vi "Exercise introduction.vi"(5 "Exercise Execution Mode":T2, 6 "Numero USP":dbl format="%#.13f", 7 "Exercise Number":T1, 8 "Error In":errorcluster, 9 "Waveform In":waveform(dbl), 10 "Array":bool[](array[boolean]), 11 "Exercise Folder Path":path) -> (0 "Error Out":errorcluster, 1 "Waveform Out":waveform(dbl), 2 "Done":dbl)   [LabVIEW 2014]
uses:
  Ctls/teval.ctl
  Ctls/t1q1.ctl
  Ctls/t1q2.ctl
  Ctls/ExerciseState.ctl
  Ctls/ExerciseNumeration.ctl
  <vilib>/Utility/miscctls.llb/LVPointTypeDef.ctl
  Ctls/radiobutton010.ctl
panel:
  out "Exercise Tab":T3(tab)
  in  "Close 3":bool
  in  "TEVAL":T4 caption="Perguntas"
  in  "Close":bool
  in  "T1E1":T5 {"C (F)" format="%#_9f"}
  in  "Close 2":bool
  in  "T1E2":T6 caption="Dado o sinal ao lado (presente no painel principal do exercício), faça uso das ferramentas até agora fornecidas para indicar:" {"C (F)" format="%#_9f"}
  # "PSI3214\nLaboratório de Instrumentação Elétrica"
  # "Avaliação do Tutorial"
  # "Ao longo do tutorial foram utilizados materiais em PDF para referência do aluno, materiais em vídeo para acompanhamento mais dinâmico. Neste questionário serão avaliados alguns parâmetros quantitativos a fim de se melhorar a qualidade dos tutoriais fornecidos ao longo dos anos. É importante deixar claro que não será pedida nenhuma informação que possa identificar o aluno, de modo a preservar a privacidade de cada um."
  # "AA.1) Em relação ao Material Escrito disponibilizado em PDF, avalie:"
  # "Muito Pequeno"
  # "Muito Grande"
  # "Pouco Tempo"
  # "Muito Tempo"
  # "Conteúdo do tutorial\npouco adequado às aulas"
  # "Conteúdo do tutorial\nbem adequado às aulas"
  # "Conteúdo do tutorial\nfoi pouco claro/coeso"
  # "Conteúdo do tutorial\nfoi bem claro/coeso"
  # "Tutorial atuou muito mal\ncomo reforço das aulas"
  # "Tutorial atuou muito bem \ncomo reforço das aulas"
  # "Problemas pouco\ncontextualizados"
  # "Problemas muito bem\ncontextualizados"
  # "Ferramentas pouco\ncontextualizadas"
  # "Ferramentas muito bem\ncontextualizadas"
  # "Foi de pouca ajuda na compreensão\nde outras materias"
  # "Foi de grande ajuda na compreensão\nde outras materias"
  # "AA.2) Em relação ao sua compreensão do tutorial, realize uma auto-avaliação sobre sua:"
  # "não compreendi nenhum tópico\nde programação apresentada"
  # "compreendi completamente\ntoda programação apresentada"
  # "não compreendi nenhum tópico\nde teoria apresentada"
  # "compreendi completamente\ntoda teoria apresentada"
  # "não compreendi nenhuma das\nproblemáticas apresentadas"
  # "compreendi completamente\ntodas as problemáticas apresentadas"
  # "PSI3214\nLaboratório de Instrumentação Elétrica"
  # "Exercício 1.1\nCircuito RC/RL"
  # "Como primeiro exercício, vamos rever como calcular parâmetros essênciais em circuitos RL/RC. Neste exercício será apresentado um circuito RL ou RC, cabe ao aluno a identificação de qual circuito se trata e como realizar os calculos dos parâmetros pedidos."
  # "Fig. 1.1 - Circuito RC"
  # "Fig. 1.2 - Circuito RL"
  # "Utilize o sinal gerado no VI [Exercicio 1.vi] para responder as perguntas abaixo:"
  # "Para fechar a tela do enunciado, pressione o botão \"Close Form\""
  # "A) Analise o sinal dado e indique:"
  # "B) Considerando as equações utilizadas para simulação de circuitos RC ou RL, dê os valores de:"
  # "PSI3214\nLaboratório de Instrumentação Elétrica"
  # "Exercício 1.2\nAcelerômetro MEMS"
  # "Até o presente momento foi realizada uma apresentação de programação em LabVIEW em vias de simular um circuito RC/RL. Na prática tal tarefa não seria de muito interesse para uma empresa. Vamos agora utilizar o ambiente LabVIEW para contextualizar a utilização de Circuitos RC/RL na industria:"
  # "Para fechar a tela do enunciado, pressione o botão \"Close Form\""
  # "Um dos grandes avanços na área de engenharia Mecânica e Elétrica das ultimas décadas é o advento das tecnologias MEMS (Sistemas Microeletromecânicos), que nos permitiu a construção de polias, engrenagens e motores em escala microscópica. Dentre algumas das microestruturas construídas podemos destacar os Acelerômetros MEMS, os quais permitiram a construção de celulares com capacidade de localização 3D, até sistemas de misseis teleguiados.\n    Vamos focar neste exercício no princípio fundamental que permite o funcionamento de um Acelerômetro MEMS. A estrutura é composta, basicamente, de um capacitor variavel. Conforme uma força é aplicada ao sensor, o eletrodo móvel se aproxima ou afasta do eletrodo fixo. Deste modo, ao medirmos a capacitância do dispositivo, mediremos indiretamente a força a ele aplicada.\n    Dentre os inúmeros modos que podemos identificar a capacitância de um circuito RC, iremos fazer uso aquele que foi utilizado ao longo do tutorial."
  # "A) Descreva o sinal de controle utilizado no sistema:"
  # "B) Com base no gráfico de corrente, indique qual a Resistência do dispositivo MEMS:"
  # "C) Com base na constante de tempo associada ao circuito, dê o valor da capacitância, C, do acelerômetro:"
  # "PSI3214\nLaboratório de Instrumentação Elétrica"
  # "Exercício 1.3\nSensor Touch"
  # "Ao longo do tutorial foram utilizados materiais em PDF para referência do aluno, materiais em vídeo para acompanhamento mais dinâmico. Neste questionário serão avaliados alguns parâmetros quantitativos a fim de se melhorar a qualidade dos tutoriais fornecidos ao longo dos anos. É importante deixar claro que não será pedida nenhuma informação que possa identificar o aluno, de modo a preservar a privacidade de cada um."
  # "PSI3214\nLaboratório de Instrumentação Elétrica"
  # "Ercercício 1.4\nMedida de Dielétrico"
  # "Ao longo do tutorial foram utilizados materiais em PDF para referência do aluno, materiais em vídeo para acompanhamento mais dinâmico. Neste questionário serão avaliados alguns parâmetros quantitativos a fim de se melhorar a qualidade dos tutoriais fornecidos ao longo dos anos. É importante deixar claro que não será pedida nenhuma informação que possa identificar o aluno, de modo a preservar a privacidade de cada um."
  # "PSI3214\nLaboratório de Instrumentação Elétrica"
  # "Exercício 1.5\nSensor de Pressão"
  # "Ao longo do tutorial foram utilizados materiais em PDF para referência do aluno, materiais em vídeo para acompanhamento mais dinâmico. Neste questionário serão avaliados alguns parâmetros quantitativos a fim de se melhorar a qualidade dos tutoriais fornecidos ao longo dos anos. É importante deixar claro que não será pedida nenhuma informação que possa identificar o aluno, de modo a preservar a privacidade de cada um."
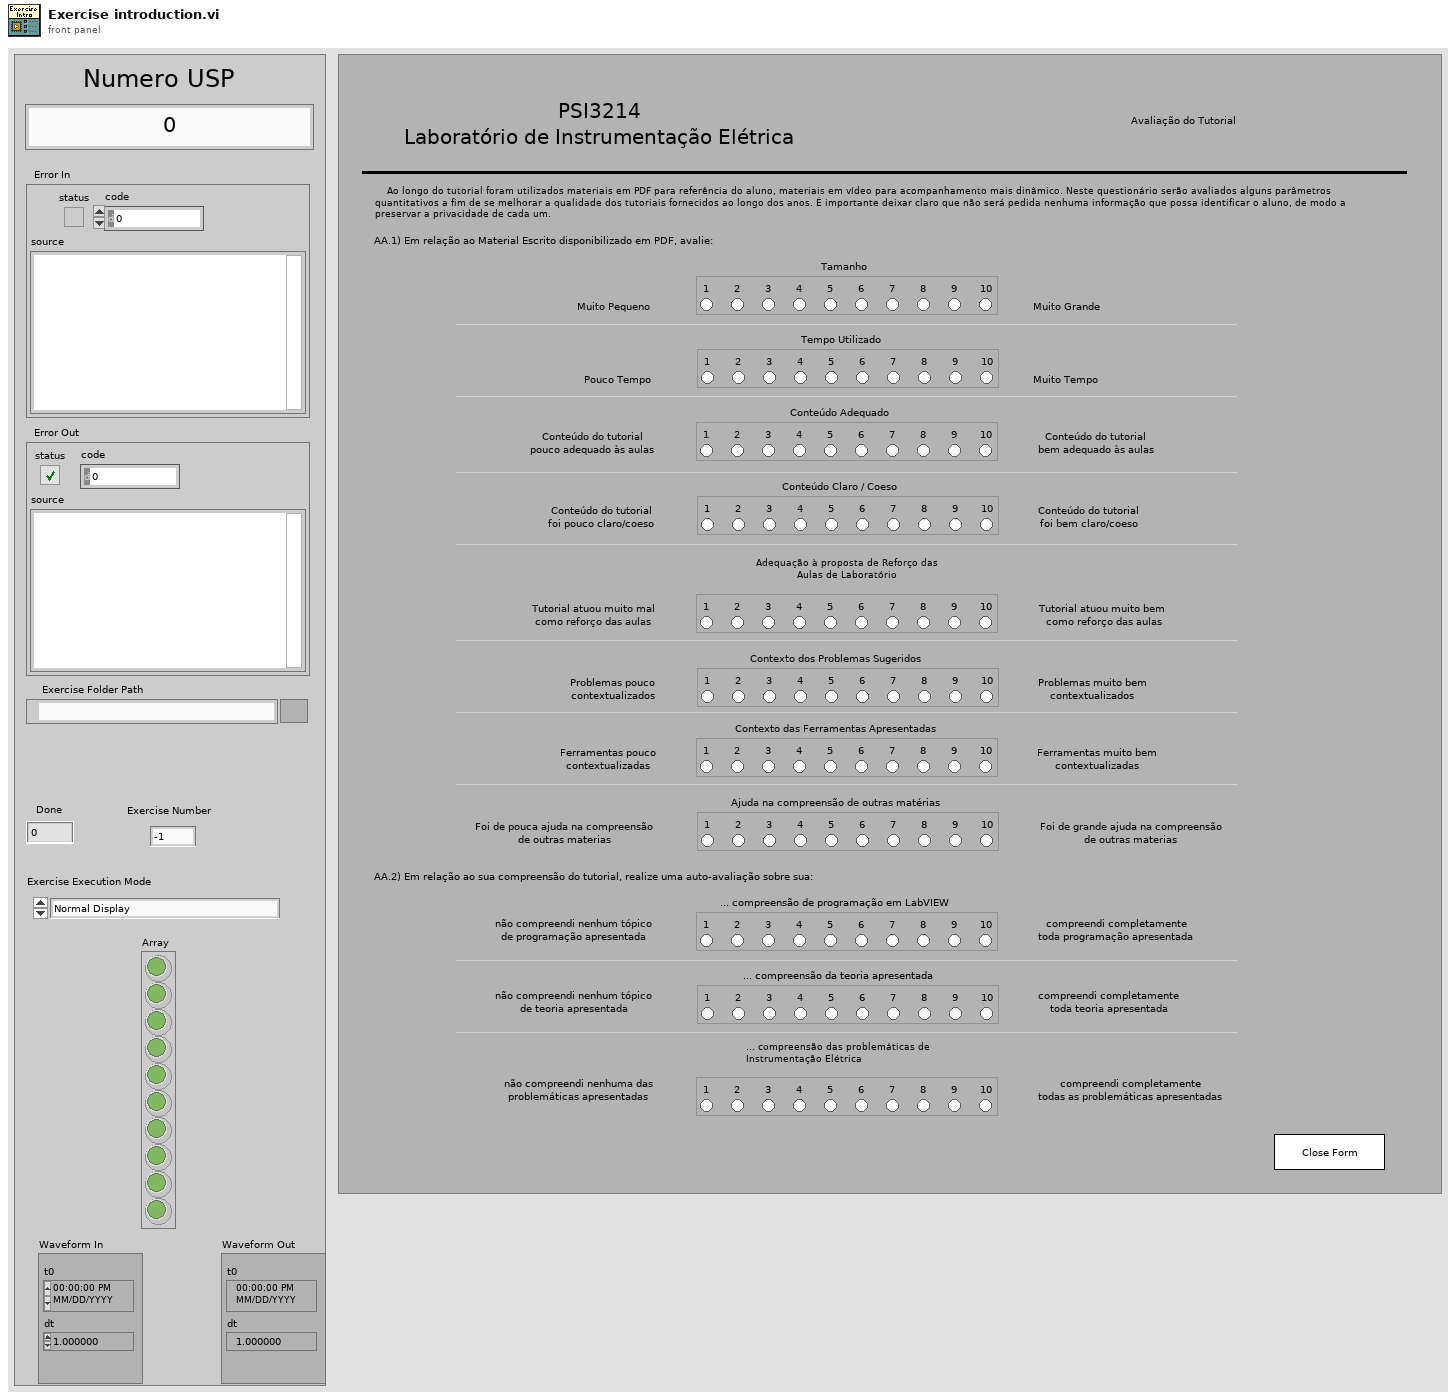
[diagram p1: front panel]
types:
  T1 = typedef "ExerciseNumeration.ctl" = enum16{"-1", "0", "1", "2", "3", "4", "5", "6", "7", "8", "9", "10"}
  T2 = typedef "ExerciseState.ctl" = enum16{"Normal Display", "Answer Highligh"}
  T3 = enum32{"Tutorial Evaluation", "Exercicio 1", "Exercicio 2", "Exercício 3", "Exercício 4", "Exercício 5"}
  T4 = typedef "teval.ctl" = cluster{"Tamanho":enum32{"No Selection", "2", "1", "3", "4", "5", "6", "7", "8", "9", "10"}, "Tempo Utilizado":enum32{"No Selection", "2", "1", "3", "4", "5", "6", "7", "8", "9", "10"}, "Conteúdo Adequado":enum32{"No Selection", "2", "1", "3", "4", "5", "6", "7", "8", "9", "10"}, "Conteúdo Claro / Coeso":enum32{"No Selection", "2", "1", "3", "4", "5", "6", "7", "8", "9", "10"}, "Adequação à proposta de Reforço das Aulas de Laboratório e de Ensino de LabVIEW":enum32{"No Selection", "2", "1", "3", "4", "5", "6", "7", "8", "9", "10"}, "Contexto dos Problemas Sugeridos":enum32{"No Selection", "2", "1", "3", "4", "5", "6", "7", "8", "9", "10"}, "Contexto das Ferramentas Apresentadas":enum32{"No Selection", "2", "1", "3", "4", "5", "6", "7", "8", "9", "10"}, "Ajuda na compreensão de outras matérias":enum32{"No Selection", "2", "1", "3", "4", "5", "6", "7", "8", "9", "10"}, "compreensão de programação em LabVIEW":enum32{"No Selection", "2", "1", "3", "4", "5", "6", "7", "8", "9", "10"}, "compreensão da teoria apresentada":enum32{"No Selection", "2", "1", "3", "4", "5", "6", "7", "8", "9", "10"}, "compreensão das problemáticas de Instrumentação Elétrica":enum32{"No Selection", "2", "1", "3", "4", "5", "6", "7", "8", "9", "10"}}
  T5 = typedef "t1q1.ctl" = cluster{"Vsig (V)":dbl, "Fsig (Hz)":dbl, "Duty Cycle (%)":dbl, "R (Ohms)":dbl, "C (F)":dbl, "L (H)":dbl, "Circuit Type":enum16{"RL", "RC"}}
  T6 = typedef "t1q2.ctl" = cluster{"Vsig (V)":dbl, "Fsig (Hz)":dbl, "R (Ohms)":dbl, "C (F)":dbl, "Duty Cycle (%)":dbl}
  T7 = typedef "LVPointTypeDef.ctl" = cluster{"Horizontal":i16, "Vertical":i16}
  T8 = enum16{"Always On", "Always Off", "Off While Running"}
  T9 = enum16{"open", "replace", "create", "open or create", "replace or create", "replace or create with confirmation"}
  T10 = typedef "radiobutton010.ctl" = enum32{"No Selection", "2", "1", "3", "4", "5", "6", "7", "8", "9", "10"}
  T11 = enum32{"No Selection", "2", "1", "3", "4", "5", "6", "7", "8", "9", "10"}
  T12 = enum32{"No Selection", "2", "1", "3", "4", "5", "6", "7", "8", "9", "10"}[]
  T13 = typedef "imagedata.ctl" = cluster{"image type":i32, "image depth":i32, "image":u8[], "mask":u8[], "colors":u32[], "Rectangle":cluster{"left":i16, "top":i16, "right":i16, "bottom":i16}}
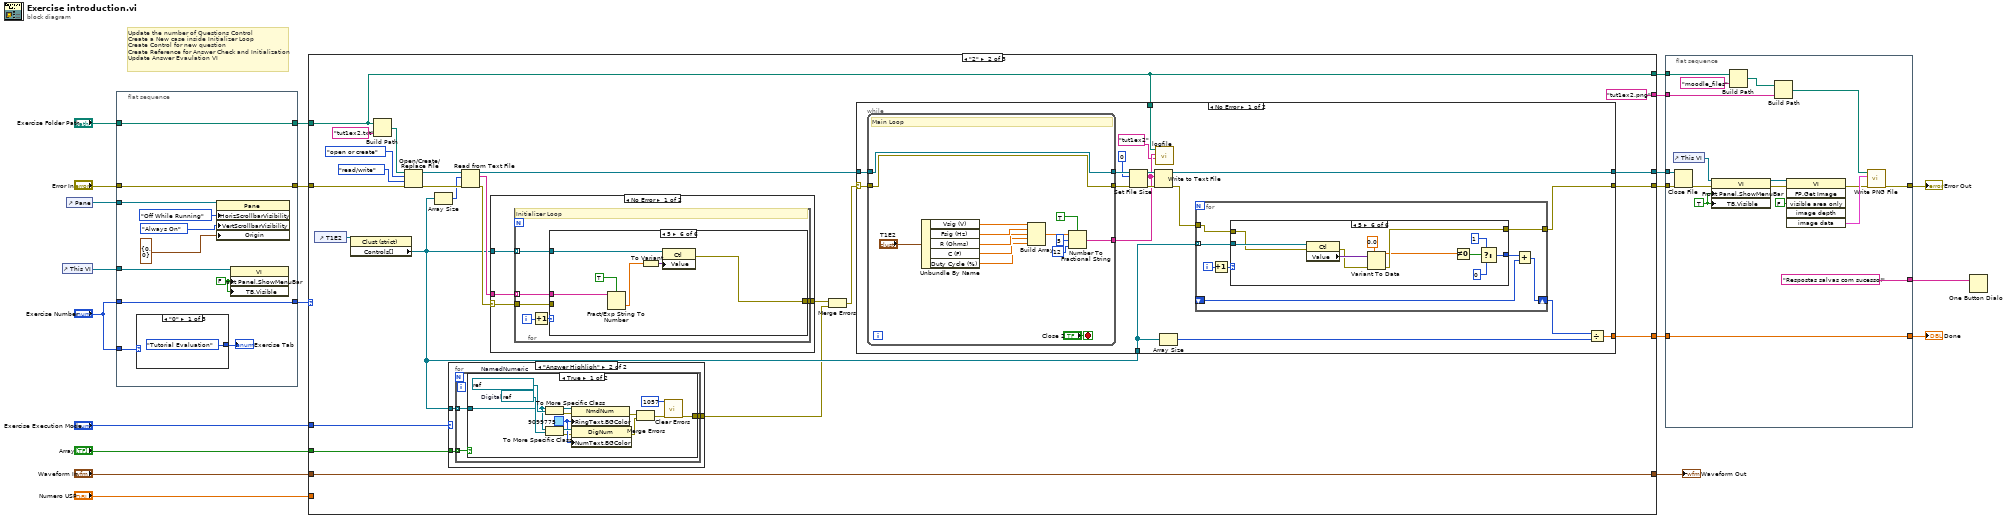
[diagram p0: block diagram]
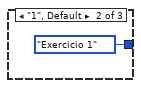
[diagram p2: hidden frame]
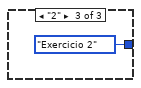
[diagram p3: hidden frame]
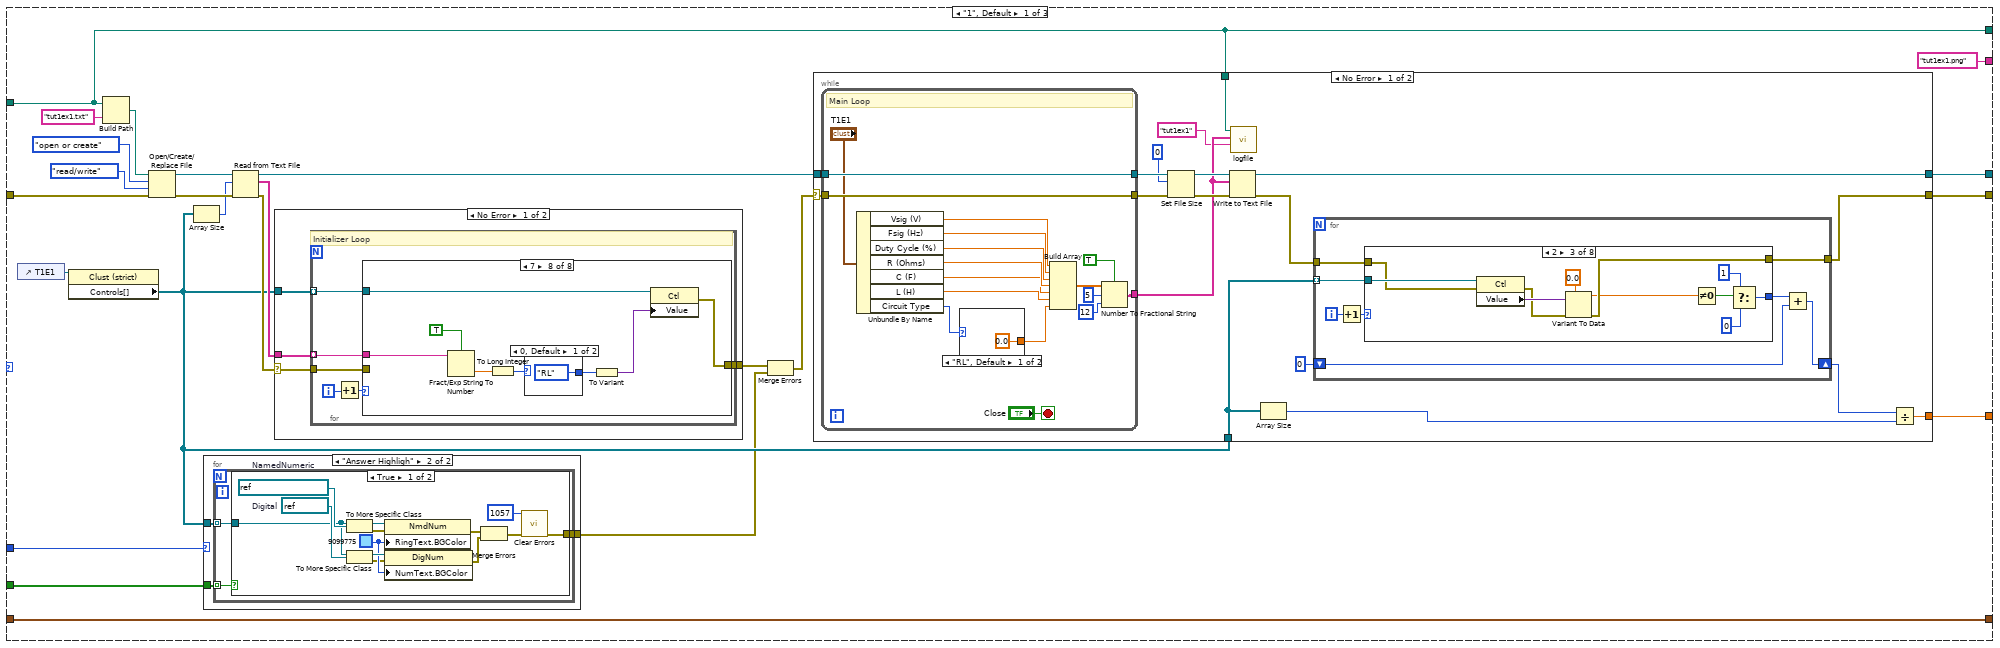
[diagram p4: hidden frame]
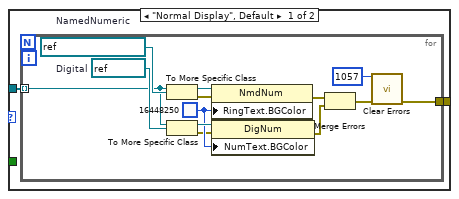
[diagram p5: hidden frame]
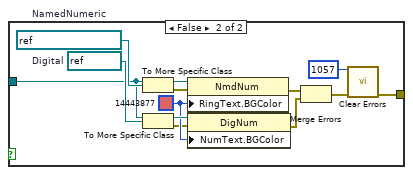
[diagram p6: hidden frame]
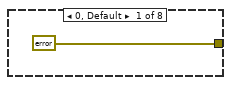
[diagram p7: hidden frame]
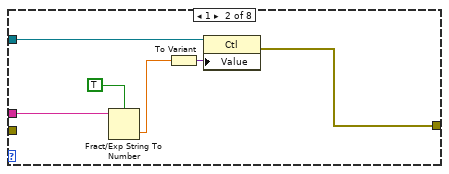
[diagram p8: hidden frame]
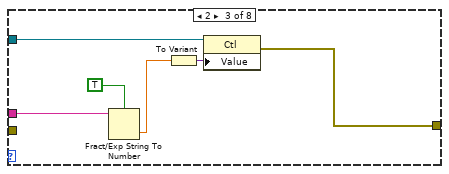
[diagram p9: hidden frame]
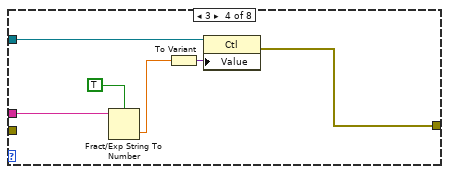
[diagram p10: hidden frame]
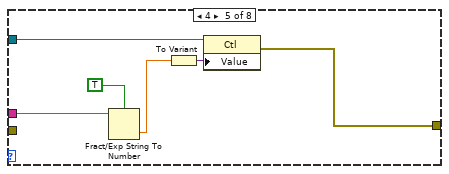
[diagram p11: hidden frame]
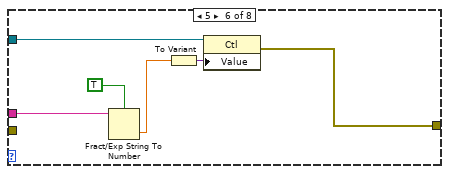
[diagram p12: hidden frame]
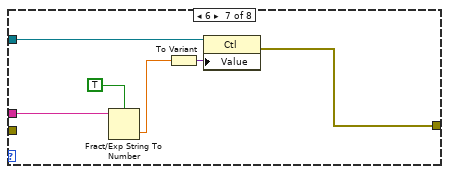
[diagram p13: hidden frame]
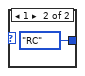
[diagram p14: hidden frame]
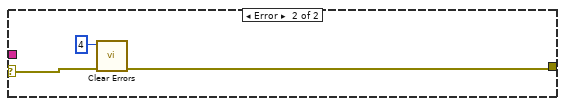
[diagram p15: hidden frame]
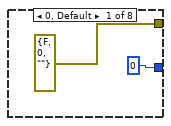
[diagram p16: hidden frame]
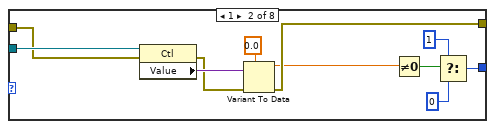
[diagram p17: hidden frame]
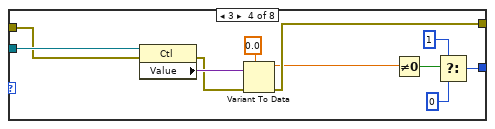
[diagram p18: hidden frame]
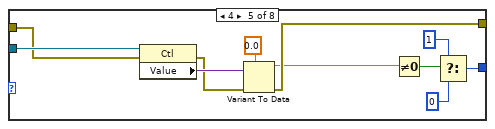
[diagram p19: hidden frame]
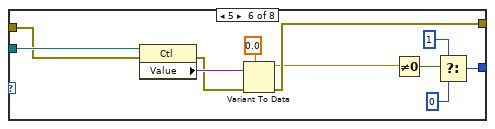
[diagram p20: hidden frame]
diagram:
  # "Update the number of Questions Control\nCreate a New case inside Initializer Loop\nCreate Control for new question\nCreate Reference for Answer Check and Initialization\nUpdate Answer Evaulation VI"
  n1 = control-ref of="This VI"() -> (w19:refnum<vi>)
  n2 = control-ref of="Pane"() -> (w10:refnum<vi>)
  n3 = flat-sequence {
    tunnel: "Exercise Number" -> [w32]
    tunnel: w10 -> [w31]
    tunnel: w19 -> [w30]
    tunnel: "Error In" -> [w26]
    tunnel: [w26] -> w17
    tunnel: "Exercise Folder Path" -> [w29]
    tunnel: [w29] -> w15
    tunnel: "Exercise Number" -> [w25]
    tunnel: [w25] -> w14
    frame #0 {
      w28 = FALSE ("Front Panel Window:Show Menu Bar")
      n4 = case shown="\"0\"" w32 {
        tunnel: [T3."Tutorial Evaluation" ("Exercise Tab") T3."Exercicio 1" ("Exercise Tab") T3."Exercicio 2" ("Exercise Tab")] -> w23
        frame "0" {
        }
        frame "1", Default {
        }
        frame "2" {
        }
      }
      "Exercise Tab" <- w23
      n5 = property class="Pane"(reference=w31, "HorizScrollbarVisibility"=T8."Off While Running" ("Horizontal Scrollbar Visibility"), "VertScrollbarVisibility"=T8."Always On" ("Vertical Scrollbar Visibility"), "Origin"=T7 {"Horizontal"=0, "Vertical"=0}) -> ()  [unwired: 1 in, 2 out]
      n6 = property class="VI"(reference=w30, "Front Panel.ShowMenuBar"=w28, "TB.Visible"=w28) -> ()  [unwired: 1 in, 2 out]
    }
  }
  n7 = case shown="\"2\"" w14 {
    tunnel: w15 -> [w36 w285 w499]
    tunnel: w17 -> [w57 w306 w516]
    tunnel: [w51 w300 w510] -> w21
    tunnel: [w50 w299 w509] -> w20
    tunnel: [w47 w296 w505] -> w11
    tunnel: "Array" -> [w43 w290 _]
    tunnel: "Exercise Execution Mode" -> [w44 w291 _]
    tunnel: "Waveform In" -> [w42 w294 w502]
    tunnel: [w42 w294 w502] -> w7
    tunnel: [w36 w285 w499] -> w4
    tunnel: ["tut1ex1.png" ("name or relative path") "tut1ex2.png" ("name or relative path") "tut1eval.png" ("name or relative path")] -> w3
    tunnel: "Numero USP" -> [_ _ _]
    frame "1", Default {
      n8 = control-ref of="T1E1"() -> (w41:refnum<vi>)
      n9 = property class="Clust (strict)"(reference=w41) -> ("Controls[]"=w45:refnum<vi>[])  [unwired: 1 in, 2 out]
      n10 = Build Path(base path=w36, name or relative path="tut1ex1.txt") -> (appended path=w58:path)
      n11 = Open/Create/Replace File(file path (use dialog)=w58, error in=w57, operation (0:open)=T9."open or create", access (0:read/write)=enum16{"read/write", "read-only", "write-only"}."read/write") -> (refnum out=w54:refnum<file>, error out=w53:errorcluster)  [unwired: 2 in, 1 out]
      n12 = Array Size(array=w45) -> (size(s)=w46:i32)
      n13 = case shown="\"Answer Highligh\"" w44 {
        tunnel: w45 -> [w61 w77]
        tunnel: w43 -> [_ w76]
        tunnel: [w60 w75] -> w39
        frame "Normal Display", Default {
          n14 = for {
            tunnel: w61 -> [w63] mode=indexing
            tunnel: [w62] -> w60
            w72 = refnum<vi> refnum  # Digital
            w73 = refnum<vi> refnum  # NamedNumeric
            w70 = u32 16448250
            n15 = To More Specific Class(target class=w73, reference=w63) -> (specific class reference=w74:refnum<vi>, error out=w67:errorcluster)  [unwired: 1 in]
            n16 = To More Specific Class(target class=w72, reference=w63) -> (specific class reference=w71:refnum<vi>, error out=w66:errorcluster)  [unwired: 1 in]
            n17 = property class="NmdNum"(reference=w74, error in=w67, "RingText.BGColor"=w70) -> (error out=w69:errorcluster)  [unwired: 1 out]
            n18 = property class="DigNum"(reference=w71, error in=w66, "NumText.BGColor"=w70) -> (error out=w68:errorcluster)  [unwired: 1 out]
            n19 = Merge Errors(w69, w68) -> (w65:errorcluster)
            n20 = call <vilib>:"Clear Errors.vi"("error in (no error)"=w65, "specific error code to clear (0: all)"=1057) -> ("error out"=w62:errorcluster)  [unwired: 4 in, 1 out]
          }
        }
        frame "Answer Highligh" {
          n21 = for {
            tunnel: w77 -> [w80] mode=indexing
            tunnel: w76 -> [w79] mode=indexing
            tunnel: [w78] -> w75
            n22 = case shown="True" w79 {
              tunnel: w80 -> [w88 w101]
              tunnel: [w82 w95] -> w78
              frame True {
                w91 = refnum<vi> refnum  # Digital
                w92 = refnum<vi> refnum  # NamedNumeric
                w89 = u32 9099775
                n23 = To More Specific Class(target class=w92, reference=w88) -> (specific class reference=w93:refnum<vi>, error out=w85:errorcluster)  [unwired: 1 in]
                n24 = To More Specific Class(target class=w91, reference=w88) -> (specific class reference=w90:refnum<vi>, error out=w84:errorcluster)  [unwired: 1 in]
                n25 = property class="NmdNum"(reference=w93, error in=w85, "RingText.BGColor"=w89) -> (error out=w87:errorcluster)  [unwired: 1 out]
                n26 = property class="DigNum"(reference=w90, error in=w84, "NumText.BGColor"=w89) -> (error out=w86:errorcluster)  [unwired: 1 out]
                n27 = Merge Errors(w87, w86) -> (w83:errorcluster)
                n28 = call <vilib>:"Clear Errors.vi"("error in (no error)"=w83, "specific error code to clear (0: all)"=1057) -> ("error out"=w82:errorcluster)  [unwired: 4 in, 1 out]
              }
              frame False {
                w104 = refnum<vi> refnum  # Digital
                w105 = refnum<vi> refnum  # NamedNumeric
                w102 = u32 14443877
                n29 = To More Specific Class(target class=w105, reference=w101) -> (specific class reference=w106:refnum<vi>, error out=w98:errorcluster)  [unwired: 1 in]
                n30 = To More Specific Class(target class=w104, reference=w101) -> (specific class reference=w103:refnum<vi>, error out=w97:errorcluster)  [unwired: 1 in]
                n31 = property class="NmdNum"(reference=w106, error in=w98, "RingText.BGColor"=w102) -> (error out=w100:errorcluster)  [unwired: 1 out]
                n32 = property class="DigNum"(reference=w103, error in=w97, "NumText.BGColor"=w102) -> (error out=w99:errorcluster)  [unwired: 1 out]
                n33 = Merge Errors(w100, w99) -> (w96:errorcluster)
                n34 = call <vilib>:"Clear Errors.vi"("error in (no error)"=w96, "specific error code to clear (0: all)"=1057) -> ("error out"=w95:errorcluster)  [unwired: 4 in, 1 out]
              }
            }
          }
        }
      }
      n35 = Read from Text File(file (use dialog)=w54, count=w46, error in=w53) -> (refnum out=w52:refnum<file>, text=w48:string[], error out=w49:errorcluster)  [unwired: 1 in, 1 out]
      n36 = case shown="No Error" w49 {
        selector: w49 -> [w109 w166]
        tunnel: w48 -> [w110 _]
        tunnel: [w108 w165] -> w40
        tunnel: w45 -> [w107 _]
        frame No Error {
          n37 = for {
            tunnel: w110 -> [w116] mode=indexing
            tunnel: [w113] -> w108
            tunnel: w109 -> [w112]
            tunnel: w107 -> [w111] mode=indexing
            i -> [w114]
            # "Initializer Loop"
            n38 = Increment(x=w114) -> (x+1=w115:i32)
            n39 = case shown="7" w115 {
              tunnel: w116 -> [_ w121 w127 w133 w139 w145 w151 w159]
              tunnel: [errorcluster {"status"=FALSE, "code"=0, "source"=""} ("error out") w123 w129 w135 w141 w147 w153 w161] -> w113
              tunnel: w112 -> [_ _ _ _ _ _ _ _]
              tunnel: w111 -> [_ w122 w128 w134 w140 w146 w152 w160]
              frame 0, Default {
              }
              frame 1 {
                n40 = Fract/Exp String To Number(use system decimal point (T)=TRUE, string=w121) -> (number=w119:dbl)  [unwired: 2 in, 1 out]
                n41 = To Variant(anything=w119) -> (Variant=w120:variant)
                n42 = property class="Ctl"(reference=w122, "Value"=w120) -> (error out=w123:errorcluster)  [unwired: 1 in, 1 out]
              }
              frame 2 {
                n43 = Fract/Exp String To Number(use system decimal point (T)=TRUE, string=w127) -> (number=w125:dbl)  [unwired: 2 in, 1 out]
                n44 = To Variant(anything=w125) -> (Variant=w126:variant)
                n45 = property class="Ctl"(reference=w128, "Value"=w126) -> (error out=w129:errorcluster)  [unwired: 1 in, 1 out]
              }
              frame 3 {
                n46 = Fract/Exp String To Number(use system decimal point (T)=TRUE, string=w133) -> (number=w131:dbl)  [unwired: 2 in, 1 out]
                n47 = To Variant(anything=w131) -> (Variant=w132:variant)
                n48 = property class="Ctl"(reference=w134, "Value"=w132) -> (error out=w135:errorcluster)  [unwired: 1 in, 1 out]
              }
              frame 4 {
                n49 = Fract/Exp String To Number(use system decimal point (T)=TRUE, string=w139) -> (number=w137:dbl)  [unwired: 2 in, 1 out]
                n50 = To Variant(anything=w137) -> (Variant=w138:variant)
                n51 = property class="Ctl"(reference=w140, "Value"=w138) -> (error out=w141:errorcluster)  [unwired: 1 in, 1 out]
              }
              frame 5 {
                n52 = Fract/Exp String To Number(use system decimal point (T)=TRUE, string=w145) -> (number=w143:dbl)  [unwired: 2 in, 1 out]
                n53 = To Variant(anything=w143) -> (Variant=w144:variant)
                n54 = property class="Ctl"(reference=w146, "Value"=w144) -> (error out=w147:errorcluster)  [unwired: 1 in, 1 out]
              }
              frame 6 {
                n55 = Fract/Exp String To Number(use system decimal point (T)=TRUE, string=w151) -> (number=w149:dbl)  [unwired: 2 in, 1 out]
                n56 = To Variant(anything=w149) -> (Variant=w150:variant)
                n57 = property class="Ctl"(reference=w152, "Value"=w150) -> (error out=w153:errorcluster)  [unwired: 1 in, 1 out]
              }
              frame 7 {
                n58 = Fract/Exp String To Number(use system decimal point (T)=TRUE, string=w159) -> (number=w154:dbl)  [unwired: 2 in, 1 out]
                n59 = To Long Integer(number=w154) -> (32bit integer=w155:i32)
                n60 = case shown="0, Default" w155 {
                  tunnel: [enum16{"RL", "RC"}."RL" ("Circuit Type") enum16{"RL", "RC"}."RC" ("Circuit Type")] -> w156
                  frame 0, Default {
                  }
                  frame 1 {
                  }
                }
                n61 = To Variant(anything=w156) -> (Variant=w158:variant)
                n62 = property class="Ctl"(reference=w160, "Value"=w158) -> (error out=w161:errorcluster)  [unwired: 1 in, 1 out]
              }
            }
          }
        }
        frame Error {
          n63 = call <vilib>:"Clear Errors.vi"("error in (no error)"=w166, "specific error code to clear (0: all)"=4) -> ("error out"=w165:errorcluster)  [unwired: 4 in, 1 out]
        }
      }
      n64 = Merge Errors(w40, w39) -> (w38:errorcluster)
      n65 = case shown="No Error" w38 {
        selector: w38 -> [w183 w283]
        tunnel: w52 -> [w184 w284]
        tunnel: [w171 w283] -> w51
        tunnel: [w182 w284] -> w50
        tunnel: [w175 -1.0] -> w47
        tunnel: w45 -> [w174 _]
        tunnel: w36 -> [w169 _]
        frame No Error {
          n66 = while {
            tunnel: w184 -> [w278]
            tunnel: w183 -> [w277]
            tunnel: [w278] -> w179
            tunnel: [w277] -> w181
            tunnel: [w272] -> w168
            stop <- "Close" stop-if-true
            # "Main Loop"
            n67 = Unbundle By Name("T1E1") -> ("Vsig (V)"=w266:dbl, "Fsig (Hz)"=w267:dbl, "Duty Cycle (%)"=w276:dbl, "R (Ohms)"=w275:dbl, "C (F)"=w274:dbl, "L (H)"=w273:dbl, "Circuit Type"=w264:enum16{"RL", "RC"})
            n68 = case shown="\"RL\", Default" w264 {
              tunnel: [0.0 ("y") 1.0 ("y")] -> w263
              frame "RL", Default {
              }
              frame "RC" {
              }
            }
            n69 = Build Array(w266, w267, w276, w275, w274, w273, w263) -> (w271:dbl[])
            n70 = Number To Fractional String(use system decimal point (T)=TRUE, number=w271, width (-)=i16 5, precision (6)=i16 12) -> (F-format string=w272:string[])
          }
          n71 = Set File Size(4:w181, 6:i64 0 ("size (in bytes)"), 7:w179) -> (0:w180:errorcluster, 3:w178:refnum<file>)
          n72 = Write to Text File(file (use dialog)=w178, text=w168, error in=w180) -> (refnum out=w182:refnum<file>, error out=w172:errorcluster)  [unwired: 1 in, 1 out]
          n73 = call "logfile.vi"("Locale"="tut1ex1" ("from"), "Text In"=w168, "Path In"=w169) -> ()  [unwired: 7 in, 2 out]
          n74 = Array Size(array=w174) -> (size(s)=w173:i32)
          n75 = for {
            shift-right: [w189] -> w176
            shift-left: 0 -> [w188]
            tunnel: w174 -> [w187] mode=indexing
            tunnel: w172 -> [w186]
            tunnel: [w185] -> w171
            i -> [w191]
            n76 = Increment(x=w191) -> (x+1=w192:i32)
            n77 = case shown="2" w192 {
              tunnel: [0 ("f") w203 w214 w225 w236 w247 w258 1 ("t")] -> w190
              tunnel: w187 -> [_ w200 w211 w222 w233 w244 w255 _]
              tunnel: w186 -> [_ w199 w210 w221 w232 w243 w254 w261]
              tunnel: [errorcluster {"status"=FALSE, "code"=0, "source"=""} ("error out") w197 w208 w219 w230 w241 w252 w261] -> w185
              frame 0, Default {
              }
              frame 1 {
                n78 = property class="Ctl"(reference=w200, error in=w199) -> (error out=w198:errorcluster, "Value"=w201:variant)  [unwired: 1 out]
                n79 = Variant To Data(error in=w198, type=0.0 ("y"), Variant=w201) -> (data=w195:dbl, error out=w197:errorcluster)
                n80 = Not Equal To 0?(x=w195) -> (x != 0?=w196:bool)
                n81 = Select(t=1, s=w196, f=0) -> (s? t:f=w203:i32)
              }
              frame 2 {
                n82 = property class="Ctl"(reference=w211, error in=w210) -> (error out=w209:errorcluster, "Value"=w212:variant)  [unwired: 1 out]
                n83 = Variant To Data(error in=w209, type=0.0 ("y"), Variant=w212) -> (data=w206:dbl, error out=w208:errorcluster)
                n84 = Not Equal To 0?(x=w206) -> (x != 0?=w207:bool)
                n85 = Select(t=1, s=w207, f=0) -> (s? t:f=w214:i32)
              }
              frame 3 {
                n86 = property class="Ctl"(reference=w222, error in=w221) -> (error out=w220:errorcluster, "Value"=w223:variant)  [unwired: 1 out]
                n87 = Variant To Data(error in=w220, type=0.0 ("y"), Variant=w223) -> (data=w217:dbl, error out=w219:errorcluster)
                n88 = Not Equal To 0?(x=w217) -> (x != 0?=w218:bool)
                n89 = Select(t=1, s=w218, f=0) -> (s? t:f=w225:i32)
              }
              frame 4 {
                n90 = property class="Ctl"(reference=w233, error in=w232) -> (error out=w231:errorcluster, "Value"=w234:variant)  [unwired: 1 out]
                n91 = Variant To Data(error in=w231, type=0.0 ("y"), Variant=w234) -> (data=w228:dbl, error out=w230:errorcluster)
                n92 = Not Equal To 0?(x=w228) -> (x != 0?=w229:bool)
                n93 = Select(t=1, s=w229, f=0) -> (s? t:f=w236:i32)
              }
              frame 5 {
                n94 = property class="Ctl"(reference=w244, error in=w243) -> (error out=w242:errorcluster, "Value"=w245:variant)  [unwired: 1 out]
                n95 = Variant To Data(error in=w242, type=0.0 ("y"), Variant=w245) -> (data=w239:dbl, error out=w241:errorcluster)
                n96 = Not Equal To 0?(x=w239) -> (x != 0?=w240:bool)
                n97 = Select(t=1, s=w240, f=0) -> (s? t:f=w247:i32)
              }
              frame 6 {
                n98 = property class="Ctl"(reference=w255, error in=w254) -> (error out=w253:errorcluster, "Value"=w256:variant)  [unwired: 1 out]
                n99 = Variant To Data(error in=w253, type=0.0 ("y"), Variant=w256) -> (data=w250:dbl, error out=w252:errorcluster)
                n100 = Not Equal To 0?(x=w250) -> (x != 0?=w251:bool)
                n101 = Select(t=1, s=w251, f=0) -> (s? t:f=w258:i32)
              }
              frame 7 {
              }
            }
            n102 = Add(x=w190, y=w188) -> (x+y=w189:i32)
          }
          n103 = Divide(x=w176, y=w173) -> (x/y=w175:dbl)
        }
        frame Error {
        }
      }
    }
    frame "2" {
      n104 = control-ref of="T1E2"() -> (w293:refnum<vi>)
      n105 = property class="Clust (strict)"(reference=w293) -> ("Controls[]"=w292:refnum<vi>[])  [unwired: 1 in, 2 out]
      n106 = Build Path(base path=w285, name or relative path="tut1ex2.txt") -> (appended path=w307:path)
      n107 = Open/Create/Replace File(file path (use dialog)=w307, error in=w306, operation (0:open)=T9."open or create", access (0:read/write)=enum16{"read/write", "read-only", "write-only"}."read/write") -> (refnum out=w303:refnum<file>, error out=w302:errorcluster)  [unwired: 2 in, 1 out]
      n108 = Array Size(array=w292) -> (size(s)=w295:i32)
      n109 = case shown="\"Answer Highligh\"" w291 {
        tunnel: w292 -> [w310 w326]
        tunnel: w290 -> [_ w325]
        tunnel: [w309 w324] -> w288
        frame "Normal Display", Default {
          n110 = for {
            tunnel: w310 -> [w312] mode=indexing
            tunnel: [w311] -> w309
            w321 = refnum<vi> refnum  # Digital
            w322 = refnum<vi> refnum  # NamedNumeric
            w319 = u32 16448250
            n111 = To More Specific Class(target class=w322, reference=w312) -> (specific class reference=w323:refnum<vi>, error out=w316:errorcluster)  [unwired: 1 in]
            n112 = To More Specific Class(target class=w321, reference=w312) -> (specific class reference=w320:refnum<vi>, error out=w315:errorcluster)  [unwired: 1 in]
            n113 = property class="NmdNum"(reference=w323, error in=w316, "RingText.BGColor"=w319) -> (error out=w318:errorcluster)  [unwired: 1 out]
            n114 = property class="DigNum"(reference=w320, error in=w315, "NumText.BGColor"=w319) -> (error out=w317:errorcluster)  [unwired: 1 out]
            n115 = Merge Errors(w318, w317) -> (w314:errorcluster)
            n116 = call <vilib>:"Clear Errors.vi"("error in (no error)"=w314, "specific error code to clear (0: all)"=1057) -> ("error out"=w311:errorcluster)  [unwired: 4 in, 1 out]
          }
        }
        frame "Answer Highligh" {
          n117 = for {
            tunnel: w326 -> [w329] mode=indexing
            tunnel: w325 -> [w328] mode=indexing
            tunnel: [w327] -> w324
            n118 = case shown="True" w328 {
              tunnel: w329 -> [w337 w350]
              tunnel: [w331 w344] -> w327
              frame True {
                w340 = refnum<vi> refnum  # Digital
                w341 = refnum<vi> refnum  # NamedNumeric
                w338 = u32 9099775
                n119 = To More Specific Class(target class=w341, reference=w337) -> (specific class reference=w342:refnum<vi>, error out=w334:errorcluster)  [unwired: 1 in]
                n120 = To More Specific Class(target class=w340, reference=w337) -> (specific class reference=w339:refnum<vi>, error out=w333:errorcluster)  [unwired: 1 in]
                n121 = property class="NmdNum"(reference=w342, error in=w334, "RingText.BGColor"=w338) -> (error out=w336:errorcluster)  [unwired: 1 out]
                n122 = property class="DigNum"(reference=w339, error in=w333, "NumText.BGColor"=w338) -> (error out=w335:errorcluster)  [unwired: 1 out]
                n123 = Merge Errors(w336, w335) -> (w332:errorcluster)
                n124 = call <vilib>:"Clear Errors.vi"("error in (no error)"=w332, "specific error code to clear (0: all)"=1057) -> ("error out"=w331:errorcluster)  [unwired: 4 in, 1 out]
              }
              frame False {
                w353 = refnum<vi> refnum  # Digital
                w354 = refnum<vi> refnum  # NamedNumeric
                w351 = u32 14443877
                n125 = To More Specific Class(target class=w354, reference=w350) -> (specific class reference=w355:refnum<vi>, error out=w347:errorcluster)  [unwired: 1 in]
                n126 = To More Specific Class(target class=w353, reference=w350) -> (specific class reference=w352:refnum<vi>, error out=w346:errorcluster)  [unwired: 1 in]
                n127 = property class="NmdNum"(reference=w355, error in=w347, "RingText.BGColor"=w351) -> (error out=w349:errorcluster)  [unwired: 1 out]
                n128 = property class="DigNum"(reference=w352, error in=w346, "NumText.BGColor"=w351) -> (error out=w348:errorcluster)  [unwired: 1 out]
                n129 = Merge Errors(w349, w348) -> (w345:errorcluster)
                n130 = call <vilib>:"Clear Errors.vi"("error in (no error)"=w345, "specific error code to clear (0: all)"=1057) -> ("error out"=w344:errorcluster)  [unwired: 4 in, 1 out]
              }
            }
          }
        }
      }
      n131 = Read from Text File(file (use dialog)=w303, count=w295, error in=w302) -> (refnum out=w301:refnum<file>, text=w297:string[], error out=w298:errorcluster)  [unwired: 1 in, 1 out]
      n132 = case shown="No Error" w298 {
        selector: w298 -> [w358 w399]
        tunnel: w297 -> [w359 _]
        tunnel: [w357 w398] -> w289
        tunnel: w292 -> [w356 _]
        frame No Error {
          n133 = for {
            tunnel: w359 -> [w362] mode=indexing
            tunnel: [w360] -> w357
            tunnel: w358 -> [w363]
            tunnel: w356 -> [w361] mode=indexing
            i -> [w365]
            # "Initializer Loop"
            n134 = Increment(x=w365) -> (x+1=w364:i32)
            n135 = case shown="5" w364 {
              tunnel: w362 -> [_ w370 w376 w382 w388 w394]
              tunnel: [errorcluster {"status"=FALSE, "code"=0, "source"=""} ("error out") w372 w378 w384 w390 w396] -> w360
              tunnel: w361 -> [_ w371 w377 w383 w389 w395]
              tunnel: w363 -> [_ _ _ _ _ _]
              frame 0, Default {
              }
              frame 1 {
                n136 = Fract/Exp String To Number(use system decimal point (T)=TRUE, string=w370) -> (number=w368:dbl)  [unwired: 2 in, 1 out]
                n137 = To Variant(anything=w368) -> (Variant=w369:variant)
                n138 = property class="Ctl"(reference=w371, "Value"=w369) -> (error out=w372:errorcluster)  [unwired: 1 in, 1 out]
              }
              frame 2 {
                n139 = Fract/Exp String To Number(use system decimal point (T)=TRUE, string=w376) -> (number=w374:dbl)  [unwired: 2 in, 1 out]
                n140 = To Variant(anything=w374) -> (Variant=w375:variant)
                n141 = property class="Ctl"(reference=w377, "Value"=w375) -> (error out=w378:errorcluster)  [unwired: 1 in, 1 out]
              }
              frame 3 {
                n142 = Fract/Exp String To Number(use system decimal point (T)=TRUE, string=w382) -> (number=w380:dbl)  [unwired: 2 in, 1 out]
                n143 = To Variant(anything=w380) -> (Variant=w381:variant)
                n144 = property class="Ctl"(reference=w383, "Value"=w381) -> (error out=w384:errorcluster)  [unwired: 1 in, 1 out]
              }
              frame 4 {
                n145 = Fract/Exp String To Number(use system decimal point (T)=TRUE, string=w388) -> (number=w386:dbl)  [unwired: 2 in, 1 out]
                n146 = To Variant(anything=w386) -> (Variant=w387:variant)
                n147 = property class="Ctl"(reference=w389, "Value"=w387) -> (error out=w390:errorcluster)  [unwired: 1 in, 1 out]
              }
              frame 5 {
                n148 = Fract/Exp String To Number(use system decimal point (T)=TRUE, string=w394) -> (number=w392:dbl)  [unwired: 2 in, 1 out]
                n149 = To Variant(anything=w392) -> (Variant=w393:variant)
                n150 = property class="Ctl"(reference=w395, "Value"=w393) -> (error out=w396:errorcluster)  [unwired: 1 in, 1 out]
              }
            }
          }
        }
        frame Error {
          n151 = call <vilib>:"Clear Errors.vi"("error in (no error)"=w399, "specific error code to clear (0: all)"=4) -> ("error out"=w398:errorcluster)  [unwired: 4 in, 1 out]
        }
      }
      n152 = Merge Errors(w289, w288) -> (w287:errorcluster)
      n153 = case shown="No Error" w287 {
        selector: w287 -> [w415 w497]
        tunnel: w301 -> [w416 w498]
        tunnel: [w403 w497] -> w300
        tunnel: [w414 w498] -> w299
        tunnel: [w407 -1.0] -> w296
        tunnel: w292 -> [w406 _]
        tunnel: w285 -> [w401 _]
        frame No Error {
          n154 = while {
            tunnel: w416 -> [w495]
            tunnel: w415 -> [w494]
            tunnel: [w495] -> w411
            tunnel: [w494] -> w413
            tunnel: [w484] -> w402
            stop <- "Close 2" stop-if-true
            # "Main Loop"
            n155 = Unbundle By Name("T1E2") -> ("Vsig (V)"=w492:dbl, "Fsig (Hz)"=w491:dbl, "R (Ohms)"=w490:dbl, "C (F)"=w489:dbl, "Duty Cycle (%)"=w488:dbl)
            n156 = Build Array(w492, w491, w490, w489, w488) -> (w483:dbl[])
            n157 = Number To Fractional String(use system decimal point (T)=TRUE, number=w483, width (-)=i16 5, precision (6)=i16 12) -> (F-format string=w484:string[])
          }
          n158 = Set File Size(4:w413, 6:i64 0 ("size (in bytes)"), 7:w411) -> (0:w412:errorcluster, 3:w410:refnum<file>)
          n159 = Write to Text File(file (use dialog)=w410, text=w402, error in=w412) -> (refnum out=w414:refnum<file>, error out=w404:errorcluster)  [unwired: 1 in, 1 out]
          n160 = call "logfile.vi"("Locale"="tut1ex2" ("from"), "Text In"=w402, "Path In"=w401) -> ()  [unwired: 7 in, 2 out]
          n161 = Array Size(array=w406) -> (size(s)=w405:i32)
          n162 = for {
            shift-right: [w423] -> w408
            shift-left: _ -> [w422]
            tunnel: w406 -> [w420] mode=indexing
            tunnel: w404 -> [w419]
            tunnel: [w417] -> w403
            i -> [w424]
            n163 = Increment(x=w424) -> (x+1=w421:i32)
            n164 = case shown="5" w421 {
              tunnel: [0 ("f") w435 w446 w457 w468 w479] -> w418
              tunnel: w420 -> [_ w432 w443 w454 w465 w476]
              tunnel: w419 -> [_ w431 w442 w453 w464 w475]
              tunnel: [errorcluster {"status"=FALSE, "code"=0, "source"=""} ("error out") w429 w440 w451 w462 w473] -> w417
              frame 0, Default {
              }
              frame 1 {
                n165 = property class="Ctl"(reference=w432, error in=w431) -> (error out=w430:errorcluster, "Value"=w433:variant)  [unwired: 1 out]
                n166 = Variant To Data(error in=w430, type=0.0 ("y"), Variant=w433) -> (data=w427:dbl, error out=w429:errorcluster)
                n167 = Not Equal To 0?(x=w427) -> (x != 0?=w428:bool)
                n168 = Select(t=1, s=w428, f=0) -> (s? t:f=w435:i32)
              }
              frame 2 {
                n169 = property class="Ctl"(reference=w443, error in=w442) -> (error out=w441:errorcluster, "Value"=w444:variant)  [unwired: 1 out]
                n170 = Variant To Data(error in=w441, type=0.0 ("y"), Variant=w444) -> (data=w438:dbl, error out=w440:errorcluster)
                n171 = Not Equal To 0?(x=w438) -> (x != 0?=w439:bool)
                n172 = Select(t=1, s=w439, f=0) -> (s? t:f=w446:i32)
              }
              frame 3 {
                n173 = property class="Ctl"(reference=w454, error in=w453) -> (error out=w452:errorcluster, "Value"=w455:variant)  [unwired: 1 out]
                n174 = Variant To Data(error in=w452, type=0.0 ("y"), Variant=w455) -> (data=w449:dbl, error out=w451:errorcluster)
                n175 = Not Equal To 0?(x=w449) -> (x != 0?=w450:bool)
                n176 = Select(t=1, s=w450, f=0) -> (s? t:f=w457:i32)
              }
              frame 4 {
                n177 = property class="Ctl"(reference=w465, error in=w464) -> (error out=w463:errorcluster, "Value"=w466:variant)  [unwired: 1 out]
                n178 = Variant To Data(error in=w463, type=0.0 ("y"), Variant=w466) -> (data=w460:dbl, error out=w462:errorcluster)
                n179 = Not Equal To 0?(x=w460) -> (x != 0?=w461:bool)
                n180 = Select(t=1, s=w461, f=0) -> (s? t:f=w468:i32)
              }
              frame 5 {
                n181 = property class="Ctl"(reference=w476, error in=w475) -> (error out=w474:errorcluster, "Value"=w477:variant)  [unwired: 1 out]
                n182 = Variant To Data(error in=w474, type=0.0 ("y"), Variant=w477) -> (data=w471:dbl, error out=w473:errorcluster)
                n183 = Not Equal To 0?(x=w471) -> (x != 0?=w472:bool)
                n184 = Select(t=1, s=w472, f=0) -> (s? t:f=w479:i32)
              }
            }
            n185 = Add(x=w418, y=w422) -> (x+y=w423:i32)
          }
          n186 = Divide(x=w408, y=w405) -> (x/y=w407:dbl)
        }
        frame Error {
        }
      }
    }
    frame "0" {
      n187 = control-ref of="TEVAL"() -> (w501:refnum<vi>)
      n188 = property class="Clust (strict)"(reference=w501) -> ("Controls[]"=w503:refnum<vi>[])  [unwired: 1 in, 2 out]
      n189 = Build Path(base path=w499, name or relative path="teval.txt") -> (appended path=w517:path)
      n190 = Open/Create/Replace File(file path (use dialog)=w517, error in=w516, operation (0:open)=T9."open or create", access (0:read/write)=enum16{"read/write", "read-only", "write-only"}."read/write") -> (refnum out=w513:refnum<file>, error out=w512:errorcluster)  [unwired: 2 in, 1 out]
      n191 = Array Size(array=w503) -> (size(s)=w504:i32)
      n192 = Read from Text File(file (use dialog)=w513, count=w504, error in=w512) -> (refnum out=w511:refnum<file>, text=w507:string[], error out=w508:errorcluster)  [unwired: 1 in, 1 out]
      n193 = case shown="No Error" w508 {
        selector: w508 -> [w521 w563]
        tunnel: w507 -> [w522 _]
        tunnel: [w520 w562] -> w506
        tunnel: w503 -> [w519 _]
        frame No Error {
          n194 = for {
            tunnel: w522 -> [w532] mode=indexing
            tunnel: [w531] -> w520
            tunnel: w521 -> [w530]
            tunnel: w519 -> [w529] mode=indexing
            # "Initializer Loop"
            n195 = Scan From String(format string="%d", input string=w532, error in=w530) -> (error out=w527:errorcluster, output 1=w525:i32)  [unwired: 2 in, 2 out]
            n196 = To Unsigned Long Integer(number=w525) -> (unsigned 32bit integer=w526:u32)
            n197 = case shown="No Error" w527 {
              selector: w527 -> [w534 w559]
              tunnel: w526 -> [w536 _]
              tunnel: [w535 radiobutton010."2" ("Radio Buttons")] -> w524
              tunnel: [w533 w559] -> w523
              frame No Error {
                n198 = case shown="0, Default" w536 {
                  tunnel: [radiobutton010."No Selection" ("Radio Buttons") radiobutton010."1" ("Radio Buttons") radiobutton010."2" ("Radio Buttons") radiobutton010."3" ("Radio Buttons") radiobutton010."4" ("Radio Buttons") radiobutton010."5" ("Radio Buttons") radiobutton010."6" ("Radio Buttons") radiobutton010."7" ("Radio Buttons") radiobutton010."8" ("Radio Buttons") radiobutton010."9" ("Radio Buttons") radiobutton010."10" ("Radio Buttons")] -> w535
                  tunnel: w534 -> [w537 w540 w542 w544 w546 w548 w550 w552 w554 w556 w558]
                  tunnel: [w537 w540 w542 w544 w546 w548 w550 w552 w554 w556 w558] -> w533
                  frame 0, Default {
                  }
                  frame 1 {
                  }
                  frame 2 {
                  }
                  frame 3 {
                  }
                  frame 4 {
                  }
                  frame 5 {
                  }
                  frame 6 {
                  }
                  frame 7 {
                  }
                  frame 8 {
                  }
                  frame 9 {
                  }
                  frame 10 {
                  }
                }
              }
              frame Error {
              }
            }
            n199 = property class="Ctl"(reference=w529, error in=w523, "Val(Sgnl)"=w524) -> (error out=w531:errorcluster)  [unwired: 1 out]
          }
        }
        frame Error {
          n200 = call <vilib>:"Clear Errors.vi"("error in (no error)"=w563, "specific error code to clear (0: all)"=4) -> ("error out"=w562:errorcluster)  [unwired: 4 in, 1 out]
        }
      }
      n201 = case shown="No Error" w506 {
        selector: w506 -> [w579 w613]
        tunnel: w511 -> [w580 w614]
        tunnel: [w567 w613] -> w510
        tunnel: [w578 w614] -> w509
        tunnel: [w571 -1.0] -> w505
        tunnel: w503 -> [w570 _]
        tunnel: w499 -> [w566 _]
        frame No Error {
          n202 = while {
            tunnel: w580 -> [w611]
            tunnel: w579 -> [w610]
            tunnel: [w611] -> w575
            tunnel: [w610] -> w577
            tunnel: [w596] -> w565
            stop <- "Close 3" stop-if-true
            # "Main Loop"
            n203 = Unbundle By Name("TEVAL") -> ("Tamanho"=w609:T11, "Tempo Utilizado"=w608:T11, "Conteúdo Adequado"=w607:T11, "Conteúdo Claro / Coeso"=w606:T11, "Adequação à proposta de Reforço das Aulas de Laboratório e de Ensino de LabVIEW"=w605:T11, "Contexto dos Problemas Sugeridos"=w604:T11, "Contexto das Ferramentas Apresentadas"=w603:T11, "Ajuda na compreensão de outras matérias"=w602:T11, "compreensão de programação em LabVIEW"=w601:T11, "compreensão da teoria apresentada"=w600:T11, "compreensão das problemáticas de Instrumentação Elétrica"=w599:T11)
            n204 = Build Array(w609, w608, w607, w606, w605, w604, w603, w602, w601, w600, w599) -> (w598:T12)
            n205 = Number To Decimal String(number=w598, width (-)=i16 2) -> (decimal integer string=w596:string[])
          }
          n206 = Set File Size(4:w577, 6:i64 0 ("size (in bytes)"), 7:w575) -> (0:w576:errorcluster, 3:w574:refnum<file>)
          n207 = Write to Text File(file (use dialog)=w574, text=w565, error in=w576) -> (refnum out=w578:refnum<file>, error out=w568:errorcluster)  [unwired: 1 in, 1 out]
          n208 = call "logfile.vi"("Locale"="tut1eval" ("from"), "Text In"=w565, "Path In"=w566) -> ()  [unwired: 7 in, 2 out]
          n209 = for {
            shift-right: [w592] -> w572
            shift-left: _ -> [w591]
            tunnel: w570 -> [w590] mode=indexing
            tunnel: w568 -> [w589]
            tunnel: [w588] -> w567
            w583 = radiobutton010."No Selection" ("y")
            # "Check for Valid Response"
            n210 = property class="Ctl"(reference=w590, error in=w589) -> (error out=w581:errorcluster, "Value"=w584:variant)  [unwired: 1 out]
            n211 = Variant To Data(error in=w581, type=w583, Variant=w584) -> (data=w582:T10, error out=w588:errorcluster)
            n212 = Not Equal?(x=w582, y=w583) -> (x != y?=w587:bool)
            n213 = Select(t=1, s=w587, f=0) -> (s? t:f=w593:i32)
            n214 = Add(x=w593, y=w591) -> (x+y=w592:i32)
          }
          n215 = Array Size(array=w570) -> (size(s)=w569:i32)
          n216 = Divide(x=w572, y=w569) -> (x/y=w571:dbl)
        }
        frame Error {
        }
      }
    }
  }
  "Waveform Out" <- w7
  n217 = flat-sequence {
    tunnel: w21 -> [w632]
    tunnel: w20 -> [w631]
    tunnel: [w621] -> w13
    tunnel: [w628] -> w12
    tunnel: w11 -> [w628]
    tunnel: w4 -> [w616]
    tunnel: w3 -> [w620]
    tunnel: ["Respostas salvas com sucesso!" ("message")] -> w2
    frame #0 {
      w630 = TRUE ("Front Panel Window:Show Menu Bar")
      n218 = control-ref of="This VI"() -> (w627:refnum<vi>)
      n219 = Close File(refnum=w631, error in=w632) -> (error out=w629:errorcluster)  [unwired: 1 out]
      n220 = property class="VI"(reference=w627, error in=w629, "Front Panel.ShowMenuBar"=w630, "TB.Visible"=w630) -> (reference out=w624:refnum<vi>, error out=w623:errorcluster)
      n221 = Build Path(base path=w616, name or relative path="moodle_files") -> (appended path=w617:path)
      n222 = Build Path(base path=w617, name or relative path=w620) -> (appended path=w619:path)
      n223 = invoke class="VI" method="FP.Get Image"(reference=w624, error in=w623, "visible area only"=FALSE ("Visible Area Only")) -> (error out=w622:errorcluster, "image data"=w625:T13)  [unwired: 3 in, 4 out]
      n224 = call <vilib>:"Write PNG File.vi"("error in (no error)"=w622, "image data"=w625, "path to PNG file"=w619) -> ("error out"=w621:errorcluster)  [unwired: 7 in, 1 out]
    }
  }
  n225 = One Button Dialog(message=w2) -> ()  [unwired: 1 in, 1 out]
  "Error Out" <- w13
  "Done" <- w12
